vi "Pulsed Current_HV Load Test_Spin2_Controller.vi"(5 "Published_Data_ID":string="HV39_", 10 "HV_Load_Steps_uA":dbl[](array[numeric])=[0.0, 5.0, 8.0, 10.0] format="%#_6p", 11 "Semiconductor Module Context":T2) -> (0 "error out":errorcluster)   [LabVIEW 2013]
uses:
  <vilib>/NI_TestStand_SemiconductorModule/NI_TestStand_Semiconductor_Module.lvlibp
  <vilib>/NI_TestStand_SemiconductorModule/NI_TestStand_Semiconductor_Module.lvlibp/PinMap/DC Power/PinsToNIDCPowerSessions.vi
  <instrlib>/niDCPower/nidcpower.llb/niDCPower Wait For Event - Event.ctl
  <vilib>/NI_TestStand_SemiconductorModule/NI_TestStand_Semiconductor_Module.lvlibp/PinMap/Deprecated/PublishDataDoubleMultiplePinsSingleInstrument.vi
  <vilib>/NI_TestStand_SemiconductorModule/NI_TestStand_Semiconductor_Module.lvlibp/PinMap/General/SemiconductorModuleContext.ctl
  Controls/Current_Pulse_Parameters.ctl
panel:
  out "Pulse_Current_Setting":dbl[](array[numeric])
  in  "Current_Pulse_Parameters":T1={"Source Delay (Sec)"=0.0, "Pulse On Time (Sec)"=0.001, "Pulse Bias Delay (Sec)"=0.0, "Aperture Time (Sec)"=1.25e-05, "Pulse Off Time (Sec)"=5e-05, "Pulse Current Level Range"=0.0001, "Pulse Bias Current Level"=0.0, "Pulse Voltage Limit"=60.0, "Pulse Voltage Limit Range"=60.0, "Pulse Bias Voltage Limit"=60.0, "Pulse Current Level"=-2.4e-05} {"Pulse Current Level" format="%.5p"; "Pulse Bias Voltage Limit" format="%.5p"; "Pulse Voltage Limit Range" format="%#.6p"; "Pulse Voltage Limit" format="%.5p"; "Pulse Bias Current Level" format="%.5p"; "Pulse Current Level Range" format="%#.6p"; "Pulse Off Time (Sec)" format="%#_6p"; "Aperture Time (Sec)" format="%#_6p"; "Pulse Bias Delay (Sec)" format="%.3p"; "Pulse On Time (Sec)" format="%#_6p"; "Source Delay (Sec)" format="%.3p"}
  out "Array 5":dbl[](array[numeric])=[40.40655357745107, 40.06989641562133, 39.73870446745766, 39.43921075855717, 39.14736834878918, 38.866456366353326, 38.60194002491567, 38.343981939877295, 38.098047324904265, 37.84446141079875, 37.56027030016325, 37.33619653985449, 37.11649495047859, 36.912095959367676, 36.70441784005712, 36.50876319081191, 36.313108541566706, 36.13275649058648, 35.95021835413984, 35.77314543135926, 35.61028206411046, 35.44632565412844, 35.28564837234606, 35.13371543242939, 34.98287553524594, 34.840779979928186, 34.69649833914401, 34.565333211158396, 34.43088895497314, 34.30081686972074, 34.17839608360084, 34.06253355388021, 33.93792668229388, 33.82862240897253, 33.718225092917976, 33.61219994779627, 33.50508175994135, 33.409987042151776]
  out "HV_V":dbl=40.06989641562133
  out "Load_Current":dbl=2.0360652503385706e-05 format="%#_6p"
  in  "Max_Load_Duration_(s)":dbl=3e-05 format="%#_6p"
  in  "Target_Load":dbl=-2e-05 format="%#_6p"
  out "Array 4":dbl[](array[numeric])=[2.0190082515575266e-05, 2.01435634279906e-05, 2.0360652503385706e-05, 2.0531222491196145e-05, 2.069293170041903e-05, 2.0841349741760583e-05, 2.091002077581414e-05, 2.1056223622508802e-05, 2.1109388294034137e-05, 2.0322994194388595e-05, 2.155907280735257e-05, 2.139736359812968e-05, 2.1514768914414793e-05, 2.1561288001999455e-05, 2.166983253969701e-05, 2.1740718768397454e-05, 2.1791668245275896e-05, 2.1869200057917007e-05, 2.1951162259851894e-05, 2.197995979026145e-05, 2.2081858744018336e-05, 2.2108441079781002e-05, 2.218597289242211e-05, 2.2239137563947445e-05, 2.227901106759144e-05, 2.2332175739116777e-05, 2.241635313569855e-05, 2.2447365860754995e-05, 2.246951780722388e-05, 2.2513821700161658e-05, 2.256698637168699e-05, 2.2613505459271655e-05, 2.2657809352209435e-05, 2.2668885325443877e-05, 2.2722049996969208e-05, 2.2770784279200764e-05, 2.281951856143232e-05, 2.2848316091841875e-05] format="%#_6p"
  out "Array 2":i32[](array[numeric])=[1, 2, 3, 4, 5, 6, 7, 8, 9, 10, 11, 12, 13, 14, 15, 16, 17, 18, 19, 20, 21, 22, 23, 24, 25, 26, 27, 28, 29, 30, 31, 32, 33, 34, 35, 36, 37, 38]
  out "Measurement:Aperture Time":dbl=1.2777777777777777e-05 format="%#_6p"
  out "Measurement:Measure Record Delta Time":dbl=1.2777777777777777e-05 format="%#_6p"
  out "Measurement:Measure Record Length":i32=39
  out "Chart_HV_Voltage":cluster{"X":dbl, "Y":dbl}[](graph)=[{"X"=0.0, "Y"=40.80551417507398}, {"X"=1.2777777777777777e-05, "Y"=40.40655357745107}, {"X"=2.5555555555555554e-05, "Y"=40.06989641562133}, {"X"=3.8333333333333334e-05, "Y"=39.73870446745766}, {"X"=5.111111111111111e-05, "Y"=39.43921075855717}, {"X"=6.388888888888888e-05, "Y"=39.14736834878918}, {"X"=7.666666666666667e-05, "Y"=38.866456366353326}, {"X"=8.944444444444444e-05, "Y"=38.60194002491567}, {"X"=0.00010222222222222222, "Y"=38.343981939877295}, {"X"=0.00011499999999999999, "Y"=38.098047324904265}, {"X"=0.00012777777777777776, "Y"=37.84446141079875}, {"X"=0.00014055555555555555, "Y"=37.56027030016325}, {"X"=0.00015333333333333334, "Y"=37.33619653985449}, {"X"=0.0001661111111111111, "Y"=37.11649495047859}, {"X"=0.00017888888888888889, "Y"=36.912095959367676}, {"X"=0.00019166666666666665, "Y"=36.70441784005712}, {"X"=0.00020444444444444443, "Y"=36.50876319081191}, {"X"=0.00021722222222222222, "Y"=36.313108541566706}, {"X"=0.00022999999999999998, "Y"=36.13275649058648}, {"X"=0.00024277777777777777, "Y"=35.95021835413984}, {"X"=0.00025555555555555553, "Y"=35.77314543135926}, {"X"=0.0002683333333333333, "Y"=35.61028206411046}, {"X"=0.0002811111111111111, "Y"=35.44632565412844}, {"X"=0.0002938888888888889, "Y"=35.28564837234606}, {"X"=0.0003066666666666667, "Y"=35.13371543242939}, {"X"=0.0003194444444444444, "Y"=34.98287553524594}, {"X"=0.0003322222222222222, "Y"=34.840779979928186}, {"X"=0.000345, "Y"=34.69649833914401}, {"X"=0.00035777777777777777, "Y"=34.565333211158396}, {"X"=0.00037055555555555556, "Y"=34.43088895497314}, {"X"=0.0003833333333333333, "Y"=34.30081686972074}, {"X"=0.0003961111111111111, "Y"=34.17839608360084}, {"X"=0.00040888888888888887, "Y"=34.06253355388021}, {"X"=0.00042166666666666665, "Y"=33.93792668229388}, {"X"=0.00043444444444444444, "Y"=33.82862240897253}, {"X"=0.00044722222222222217, "Y"=33.718225092917976}, {"X"=0.00045999999999999996, "Y"=33.61219994779627}, {"X"=0.00047277777777777775, "Y"=33.50508175994135}, {"X"=0.00048555555555555553, "Y"=33.409987042151776}]
  out "Chart_Measured_Load_Current":cluster{"X":dbl, "Y":dbl}[](graph)=[{"X"=0.0, "Y"=-1.8588496785874633e-05}, {"X"=1.2777777777777777e-05, "Y"=-2.0190082515575266e-05}, {"X"=2.5555555555555554e-05, "Y"=-2.01435634279906e-05}, {"X"=3.8333333333333334e-05, "Y"=-2.0360652503385706e-05}, {"X"=5.111111111111111e-05, "Y"=-2.0531222491196145e-05}, {"X"=6.388888888888888e-05, "Y"=-2.069293170041903e-05}, {"X"=7.666666666666667e-05, "Y"=-2.0841349741760583e-05}, {"X"=8.944444444444444e-05, "Y"=-2.091002077581414e-05}, {"X"=0.00010222222222222222, "Y"=-2.1056223622508802e-05}, {"X"=0.00011499999999999999, "Y"=-2.1109388294034137e-05}, {"X"=0.00012777777777777776, "Y"=-2.0322994194388595e-05}, {"X"=0.00014055555555555555, "Y"=-2.155907280735257e-05}, {"X"=0.00015333333333333334, "Y"=-2.139736359812968e-05}, {"X"=0.0001661111111111111, "Y"=-2.1514768914414793e-05}, {"X"=0.00017888888888888889, "Y"=-2.1561288001999455e-05}, {"X"=0.00019166666666666665, "Y"=-2.166983253969701e-05}, {"X"=0.00020444444444444443, "Y"=-2.1740718768397454e-05}, {"X"=0.00021722222222222222, "Y"=-2.1791668245275896e-05}, {"X"=0.00022999999999999998, "Y"=-2.1869200057917007e-05}, {"X"=0.00024277777777777777, "Y"=-2.1951162259851894e-05}, {"X"=0.00025555555555555553, "Y"=-2.197995979026145e-05}, {"X"=0.0002683333333333333, "Y"=-2.2081858744018336e-05}, {"X"=0.0002811111111111111, "Y"=-2.2108441079781002e-05}, {"X"=0.0002938888888888889, "Y"=-2.218597289242211e-05}, {"X"=0.0003066666666666667, "Y"=-2.2239137563947445e-05}, {"X"=0.0003194444444444444, "Y"=-2.227901106759144e-05}, {"X"=0.0003322222222222222, "Y"=-2.2332175739116777e-05}, {"X"=0.000345, "Y"=-2.241635313569855e-05}, {"X"=0.00035777777777777777, "Y"=-2.2447365860754995e-05}, {"X"=0.00037055555555555556, "Y"=-2.246951780722388e-05}, {"X"=0.0003833333333333333, "Y"=-2.2513821700161658e-05}, {"X"=0.0003961111111111111, "Y"=-2.256698637168699e-05}, {"X"=0.00040888888888888887, "Y"=-2.2613505459271655e-05}, {"X"=0.00042166666666666665, "Y"=-2.2657809352209435e-05}, {"X"=0.00043444444444444444, "Y"=-2.2668885325443877e-05}, {"X"=0.00044722222222222217, "Y"=-2.2722049996969208e-05}, {"X"=0.00045999999999999996, "Y"=-2.2770784279200764e-05}, {"X"=0.00047277777777777775, "Y"=-2.281951856143232e-05}, {"X"=0.00048555555555555553, "Y"=-2.2848316091841875e-05}]
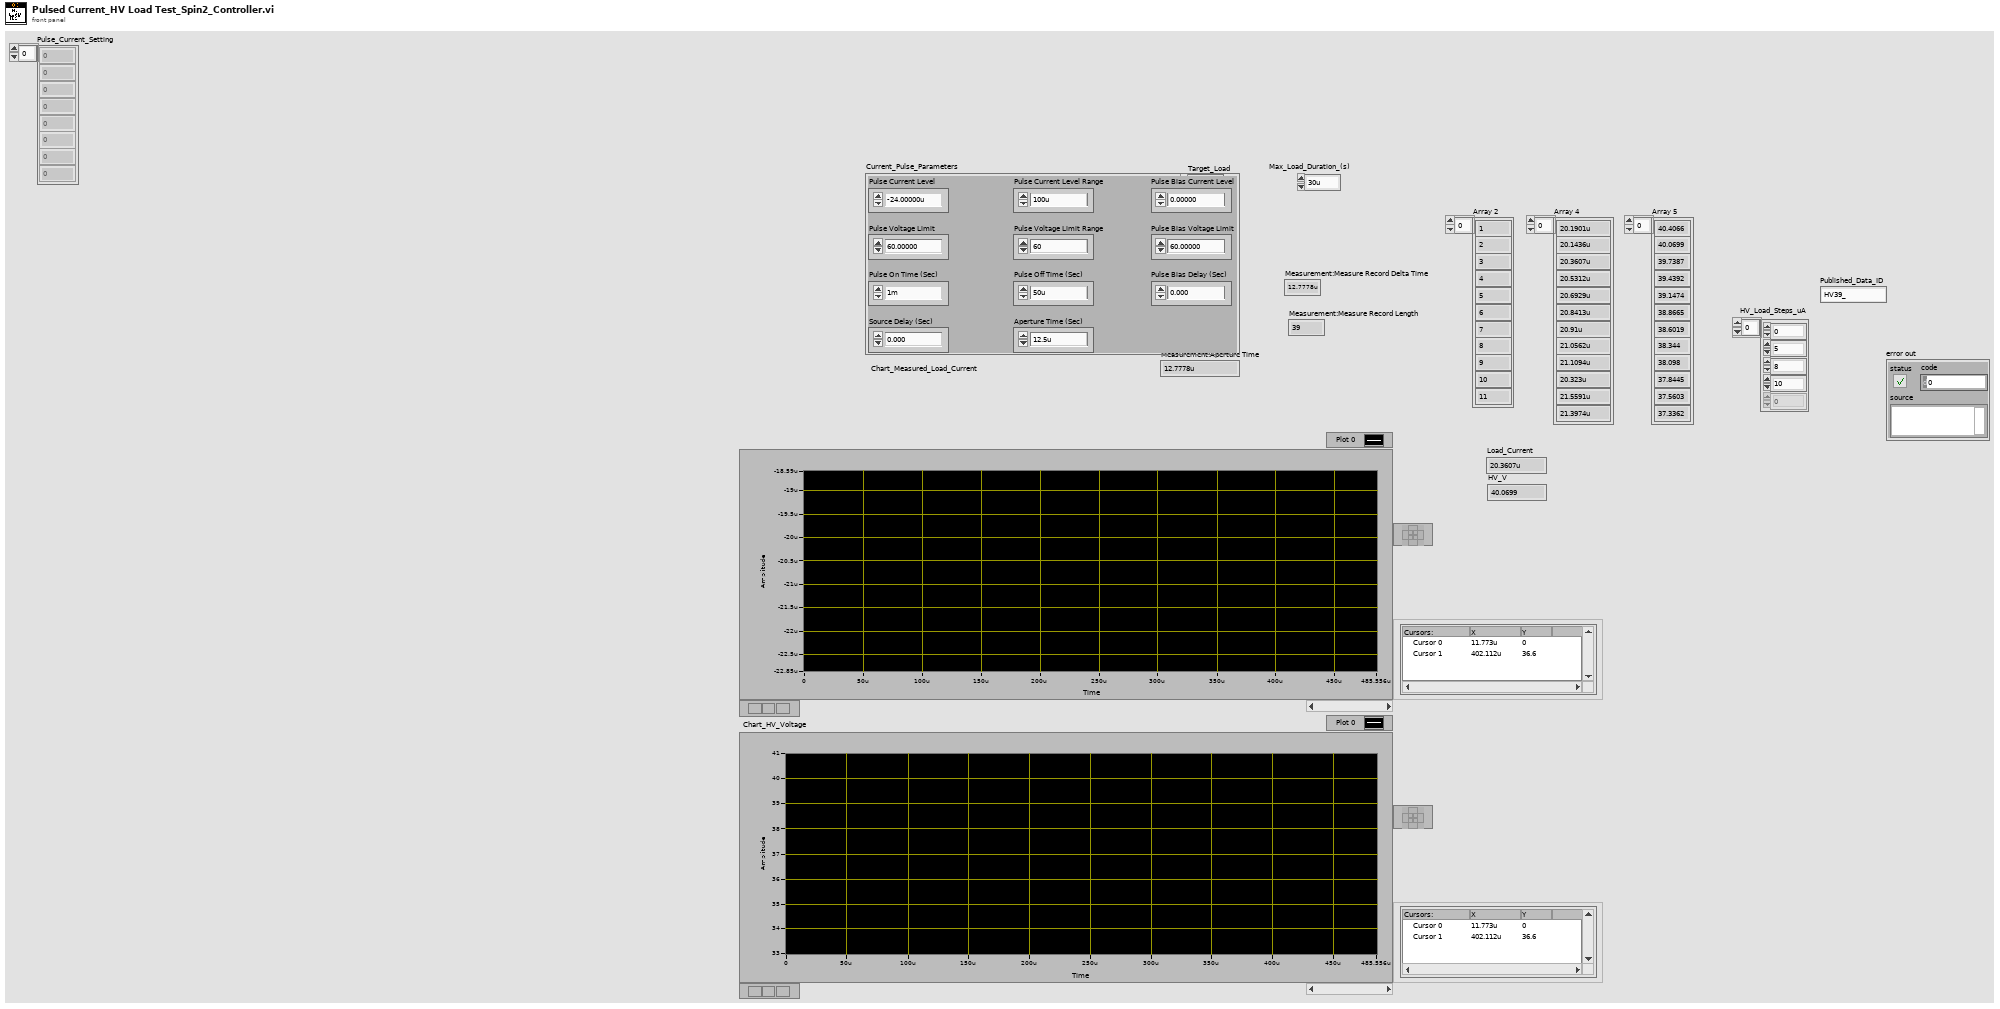
[diagram p1: front panel]
types:
  T1 = typedef "Current_Pulse_Parameters.ctl" = cluster{"Source Delay (Sec)":dbl, "Pulse On Time (Sec)":dbl, "Pulse Bias Delay (Sec)":dbl, "Aperture Time (Sec)":dbl, "Pulse Off Time (Sec)":dbl, "Pulse Current Level Range":dbl, "Pulse Bias Current Level":dbl, "Pulse Voltage Limit":dbl, "Pulse Voltage Limit Range":dbl, "Pulse Bias Voltage Limit":dbl, "Pulse Current Level":dbl}
  T2 = typedef "NI_TestStand_Semiconductor_Module.lvlibp/SemiconductorModuleContext.ctl" = refnum<k7>
  T3 = typedef "niDCPower Wait For Event - Event.ctl" = i32
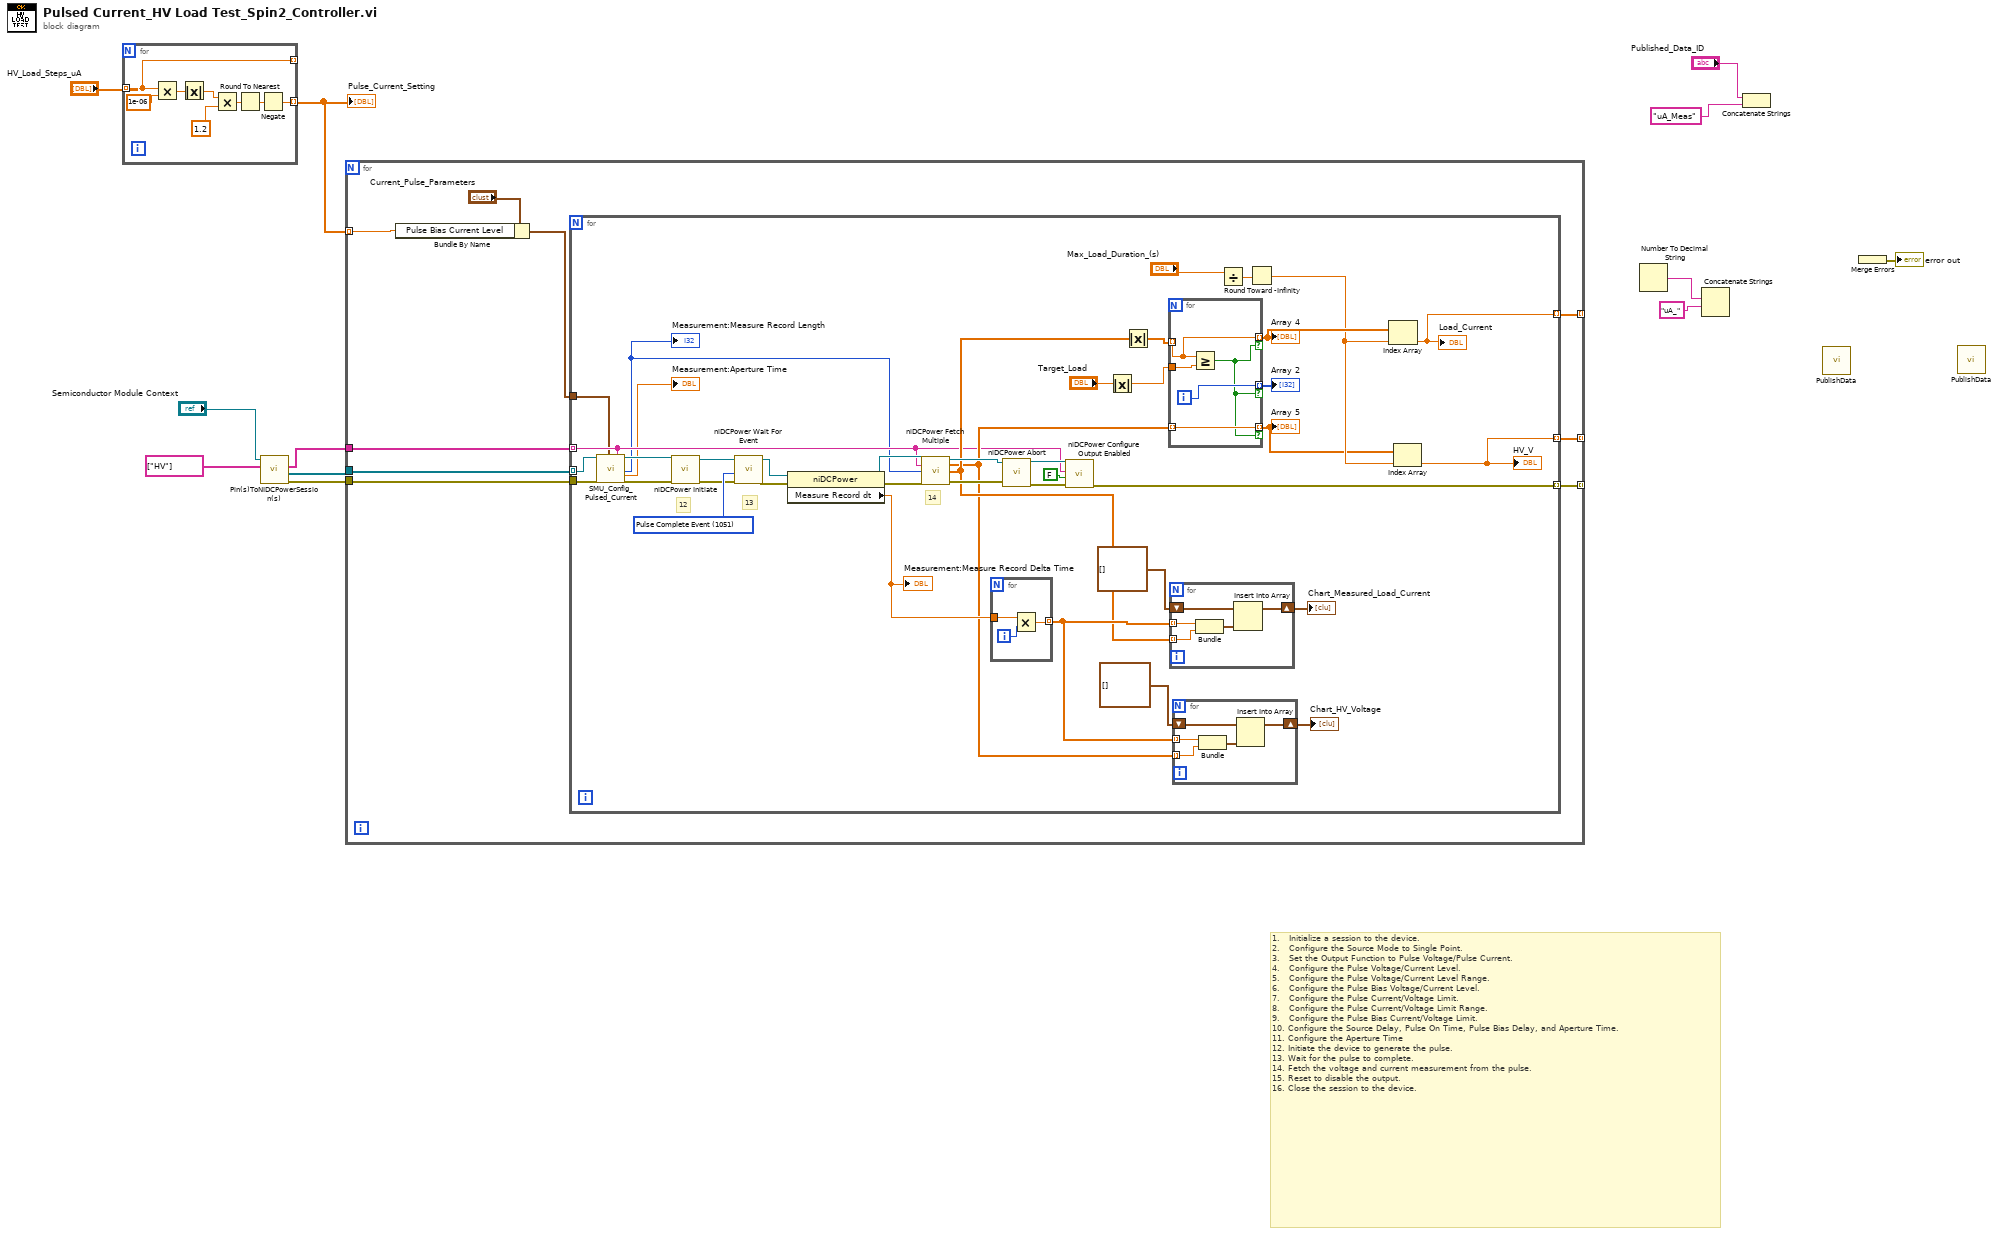
[diagram p0: block diagram]
diagram:
  # "1.   Initialize a session to the device.\n2.   Configure the Source Mode to Single Point.\n3.   Set the Output Function to Pulse Voltage/Pulse Current.\n4.   Configure the Pulse Voltage/Current Level.\n5.   Configure the Pulse Voltage/Current Level Range.\n6.   Configure the Pulse Bias Voltage/Current Level.\n7.   Configure the Pulse Current/Voltage Limit. \n8.   Configure the Pulse Current/Voltage Limit Range.\n9.   Configure the Pulse Bias Current/Voltage Limit.\n10. Configure the Source Delay, Pulse On Time, Pulse Bias Delay, and Aperture Time.\n11. Configure the Aperture Time\n12. Initiate the device to generate the pulse.\n13. Wait for the pulse to complete.\n14. Fetch the voltage and current measurement from the pulse.\n15. Reset to disable the output.\n16. Close the session to the device."
  n1 = for {
    tunnel: "HV_Load_Steps_uA" -> [w13] mode=indexing
    tunnel: [w16] -> w3 mode=indexing
    tunnel: [w13] -> _ mode=indexing
    n2 = Multiply(x=w13, y=1e-06) -> (x*y=w14:dbl)
    n3 = Absolute Value(x=w14) -> (abs(x)=w20:dbl)
    n4 = Multiply(x=w20, y=1.2) -> (x*y=w18:dbl)
    n5 = Round To Nearest(number=w18) -> (nearest integer value=w17:dbl)
    n6 = Negate(x=w17) -> (-x=w16:dbl)
  }
  "Pulse_Current_Setting" <- w3
  n7 = call-poly <vilib>:"Pin(s)ToNIDCPowerSession(s).vi"("Pins"=string[] ["HV"], "Semiconductor Module Context"="Semiconductor Module Context") -> ("error out"=w10:errorcluster, "Instrument Sessions"=w9:refnum<k15>[], "Channel Lists"=w11:string[])  [unwired: 5 in, 2 out]
  n8 = for {
    tunnel: w11 -> [w29]
    tunnel: w10 -> [w28]
    tunnel: w9 -> [w27]
    tunnel: w3 -> [w23] mode=indexing
    tunnel: [w26] -> _ mode=indexing
    tunnel: [w22] -> _ mode=indexing
    tunnel: [w21] -> _ mode=indexing
    n9 = Bundle By Name(cluster="Current_Pulse_Parameters", "Pulse Bias Current Level"=w23) -> (w24:T1)
    n10 = for {
      tunnel: w29 -> [w38] mode=indexing
      tunnel: w28 -> [w37]
      tunnel: w27 -> [w36] mode=indexing
      tunnel: w24 -> [w32]
      tunnel: [w33] -> w26 mode=indexing
      tunnel: [w31] -> w22 mode=indexing
      tunnel: [w30] -> w21 mode=indexing
      w69 = T3 1051 items=["Source Complete Event"=1030, "Measure Complete Event"=1031, "Sequence Iteration Complete Event"=1032, "Sequence Engine Done Event"=1033, "Pulse Complete Event"=1051, "Ready For Pulse Trigger Event"=1052] ("event")
      # "14"
      # "13"
      # "12"
      n11 = call "SMU_Config_Pulsed_Current.vi"("IVI Refnum in"=w36, "error in (no error)"=w37, "Current_Pulse_Parameters"=w32, "Channel List"=w38) -> ("IVI Refnum out"=w51:refnum<k15>, "Measurement:Measure Record Length"=w34:i32, "Measurement:Aperture Time"=→"Measurement:Aperture Time":dbl, "error out"=w50:errorcluster)  [unwired: 12 in]
      "Measurement:Measure Record Length" <- w34
      n12 = call <instrlib>:"niDCPower Initiate.vi"("error in (no error)"=w50, "instrument handle"=w51) -> ("error out"=w67:errorcluster, "instrument handle out"=w68:refnum<k15>)  [unwired: 2 in, 6 out]
      n13 = call <instrlib>:"niDCPower Wait For Event.vi"("error in (no error)"=w67, "event"=w69, "instrument handle"=w68) -> ("error out"=w63:errorcluster, "instrument handle out"=w64:refnum<k15>)  [unwired: 7 in]
      n14 = property class="niDCPower"(reference=w64, error in=w63) -> (reference out=w61:refnum<k15>, error out=w62:errorcluster, "Measure Record dt"=w60:dbl)
      "Measurement:Measure Record Delta Time" <- w60
      n15 = call <instrlib>:"niDCPower Fetch Multiple.vi"("instrument handle"=w61, "channel name"=w38, "count (1)"=w34, "error in (no error)"=w62) -> ("instrument handle out"=w55:refnum<k15>, "voltage measurements"=w40:dbl[], "current measurements"=w48:dbl[], "error out"=w56:errorcluster)  [unwired: 6 in, 2 out]
      n16 = for {
        tunnel: [w86] -> w57 mode=indexing
        tunnel: w60 -> [w85]
        i -> [w87]
        n17 = Multiply(x=w85, y=w87) -> (x*y=w86:dbl)
      }
      n18 = call <instrlib>:"niDCPower Abort.vi"("error in (no error)"=w56, "instrument handle"=w55) -> ("error out"=w54:errorcluster, "instrument handle out"=w53:refnum<k15>)  [unwired: 8 in]
      n19 = call <instrlib>:"niDCPower Configure Output Enabled.vi"("error in (no error)"=w54, "output enabled"=FALSE, "channel name"=w38, "instrument handle"=w53) -> ("error out"=w33:errorcluster)  [unwired: 6 in, 1 out]
      n20 = Absolute Value(x="Target_Load") -> (abs(x)=w46:dbl)
      n21 = Absolute Value(x=w48) -> (abs(x)=w47:dbl[])
      n22 = for {
        tunnel: w47 -> [w73] mode=indexing
        tunnel: w46 -> [w74]
        tunnel: [w73] -> w42 mode=indexing if=w70
        tunnel: [w72] -> w49 mode=indexing if=w70
        tunnel: w40 -> [w71] mode=indexing
        tunnel: [w71] -> w39 mode=indexing if=w70
        i -> [w72]
        n23 = Greater Or Equal?(x=w73, y=w74) -> (x >= y?=w70:bool)
      }
      "Array 2" <- w49
      "Array 4" <- w42
      "Array 5" <- w39
      n24 = for {
        shift-right: [w83] -> w65
        shift-left: cluster{"X":dbl, "Y":dbl}[] [] ("XY Graph") -> [w84]
        tunnel: w57 -> [w82] mode=indexing
        tunnel: w48 -> [w81] mode=indexing
        n25 = Bundle(w82, w81) -> (w80:cluster{dbl, dbl})  [unwired: 1 in]
        n26 = Insert Into Array(array=w84, new element=w80) -> (w83:cluster{"X":dbl, "Y":dbl}[])  [unwired: 1 in]
      }
      "Chart_Measured_Load_Current" <- w65
      n27 = for {
        shift-right: [w78] -> w58
        shift-left: cluster{"X":dbl, "Y":dbl}[] [] ("XY Graph") -> [w79]
        tunnel: w57 -> [w77] mode=indexing
        tunnel: w40 -> [w76] mode=indexing
        n28 = Bundle(w77, w76) -> (w75:cluster{dbl, dbl})  [unwired: 1 in]
        n29 = Insert Into Array(array=w79, new element=w75) -> (w78:cluster{"X":dbl, "Y":dbl}[])  [unwired: 1 in]
      }
      "Chart_HV_Voltage" <- w58
      n30 = Divide(x="Max_Load_Duration_(s)") -> (x/y=w43:dbl)  [unwired: 1 in]
      n31 = Round Toward -Infinity(1:w43) -> (0:w41:dbl)
      n32 = Index Array(array=w42, index=w41) -> (element=w31:dbl)
      "Load_Current" <- w31
      n33 = Index Array(array=w39, index=w41) -> (element=w30:dbl)
      "HV_V" <- w30
    }
  }
  n34 = Number To Decimal String() -> (decimal integer string=w6:string)  [unwired: 2 in]
  n35 = Concatenate Strings(w6, "uA_" ("string")) -> ()  [unwired: 2 in, 1 out]
  n36 = Concatenate Strings("Published_Data_ID", "uA_Meas" ("string")) -> ()  [unwired: 1 out]
  n37 = call-poly <vilib>:"PublishData.vi"() -> ()  [unwired: 10 in, 2 out]
  n38 = Merge Errors() -> (→"error out":errorcluster)  [unwired: 1 in]
  n39 = call-poly <vilib>:"PublishData.vi"() -> ()  [unwired: 10 in, 2 out]
